vi "Check New Segment.vi"(8 "error in (no error)":errorcluster, 10 "Waveform Info":T1, 11 "Waveform Buffer in":refnum<class "Waveform Buffer.lvclass">) -> (0 "error out":errorcluster, 3 "Waveform Buffer out":refnum<class "Waveform Buffer.lvclass">)   [LabVIEW 2012, in "Waveform Data Logger Engine.lvlib" / "Waveform Buffer.lvclass"]
uses:
  Waveform Buffer.lvclass
  Waveform Receive/Wfm Info.ctl
  Waveform Buffer.lvclass/Waveform Buffer.ctl
  Wfm Segment.ctl
  Data Point.ctl
  Waveform Receive/Waveform Receive.lvclass
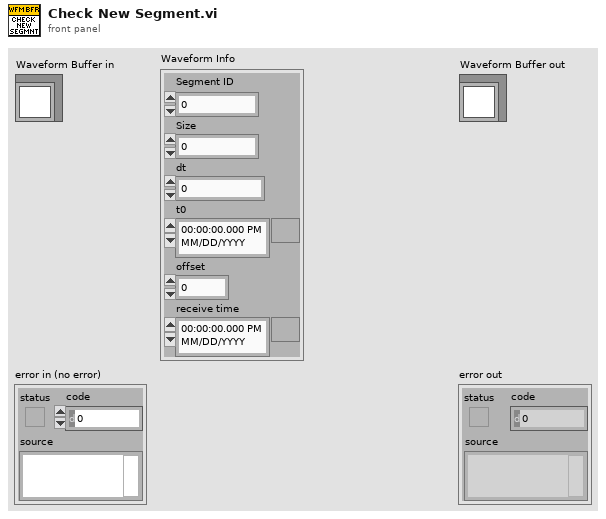
[diagram p1: front panel]
types:
  T1 = typedef "Waveform Data Logger Engine.lvlib/Waveform Receive.lvclass/Wfm Info.ctl" = cluster{"Segment ID":u64, "Size":i32, "dt":dbl, "t0":timestamp, "offset":u64, "receive time":timestamp}
  T2 = typedef "Waveform Data Logger Engine.lvlib/Waveform Buffer.lvclass/Wfm Segment.ctl" = cluster{"ID":u64, "Total samples":i32, "Start":T3, "Finish":T3}
  T3 = typedef "Waveform Data Logger Engine.lvlib/Waveform Buffer.lvclass/Data Point.ctl" = cluster{"Index":i32, "Wfm time":timestamp, "Receive time":timestamp}
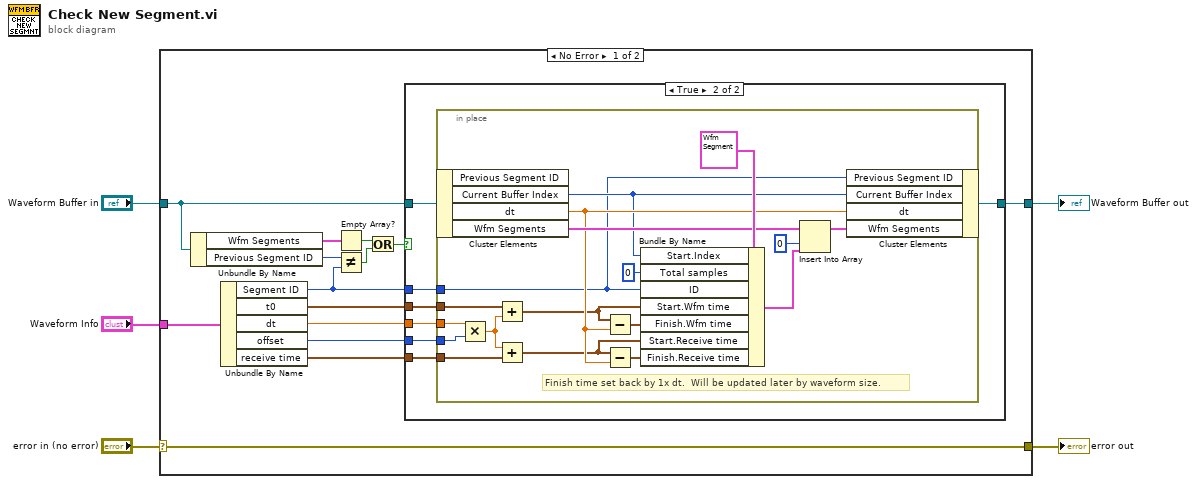
[diagram p0: block diagram]
diagram:
  n1 = case shown="No Error" "error in (no error)" {
    selector: "error in (no error)" -> [w16 w47]
    tunnel: [w16 w47] -> w4
    tunnel: [w15 w46] -> w2
    tunnel: "Waveform Buffer in" -> [w14 w46]
    tunnel: "Waveform Info" -> [w19 _]
    frame No Error {
      n2 = Unbundle By Name(w14) -> ("Wfm Segments"=w11:T2[], "Previous Segment ID"=w9:u64)
      n3 = Unbundle By Name(w19) -> ("Segment ID"=w8:u64, "t0"=w18:timestamp, "dt"=w7:dbl, "offset"=w6:u64, "receive time"=w17:timestamp)
      n4 = Empty Array?(array=w11) -> (empty?=w13:bool)
      n5 = Not Equal?(x=w9, y=w8) -> (x != y?=w10:bool)
      n6 = Or(x=w13, y=w10) -> (x .or. y?=w12:bool)
      n7 = case shown="True" w12 {
        tunnel: w14 -> [w20 w27]
        tunnel: w18 -> [_ w26]
        tunnel: w17 -> [_ w25]
        tunnel: [w20 w24] -> w15
        tunnel: w8 -> [_ w23]
        tunnel: w7 -> [_ w22]
        tunnel: w6 -> [_ w21]
        frame False {
        }
        frame True {
          n8 = in-place {
            in-place-border: w26 -> [w33]
            in-place-border: w25 -> [w30]
            in-place-border: w23 -> [w36]
            in-place-border: w22 -> [w35]
            in-place-border: w21 -> [w34]
            # "Finish time set back by 1x dt.  Will be updated later by waveform size."
            n9 = in-place-cluster #1(w27) -> ("Current Buffer Index"=w37:i32, "dt"=w38:dbl, "Wfm Segments"=w42:T2[])  [unwired: 1 out]
            n10 = Multiply(x=w35, y=w34) -> (x*y=w29:dbl)
            n11 = Add(x=w33, y=w29) -> (x+y=w32:timestamp)
            n12 = Add(x=w29, y=w30) -> (x+y=w31:timestamp)
            n13 = Subtract(x=w32, y=w38) -> (x-y=w28:timestamp)
            n14 = Subtract(x=w31, y=w38) -> (x-y=w39:timestamp)
            n15 = Bundle By Name(cluster=T2 {"ID"=0, "Total samples"=0, "Start"={"Index"=0, "Wfm time"=timestamp(0 s since 1904-01-01), "Receive time"=timestamp(0 s since 1904-01-01)}, "Finish"={"Index"=0, "Wfm time"=timestamp(0 s since 1904-01-01), "Receive time"=timestamp(0 s since 1904-01-01)}} ("Wfm Segment"), "Start.Index"=w37, "Total samples"=0, "ID"=w36, "Start.Wfm time"=w32, "Finish.Wfm time"=w28, "Start.Receive time"=w31, "Finish.Receive time"=w39) -> (w43:T2)
            n16 = Insert Into Array(array=w42, index=0, new element=w43) -> (w41:T2[])
            n17 = in-place-cluster #1("Previous Segment ID"=w36, "Current Buffer Index"=w37, "dt"=w38, "Wfm Segments"=w41) -> (w24:refnum<class "Waveform Buffer.lvclass">)
          }
        }
      }
    }
    frame Error {
    }
  }
  "error out" <- w4
  "Waveform Buffer out" <- w2
